vi "KalmanFilterExample.vi"() -> ()   [LabVIEW 2016]
uses:
  <vilib>/addons/Control Design/_Stochastic Systems/Stochastic Systems.llb/Stochastic Systems SubVIs/cd_Stochastic State-Space Model.ctl
  <vilib>/Simulation/Estimation/Implementation/NILVSim Discrete Kalman Filter.llb/SIM Disc KF Pred and Corr with Pred Gain with Checking Direct LV.vi
  <vilib>/Simulation/Implementation/XNodeFramework/SimXNode/SimX.xnode
  <vilib>/addons/Control Design/_Stochastic Systems/NI_CD_Stochastic Systems.lvlib
panel:
  in  "Numeric 2":dbl=5.0 format="%#_13g"
  out "Waveform Chart 2":dbl[](graph)
  out "Waveform Chart":dbl[](graph)
  out "Numeric":i32
  out "Corrected State Estimate xhat(k|k)":dbl[](array[numeric])
  out "Estimated Output yhat(k)":dbl[](array[numeric])
  out "error out":errorcluster
  in  "stop":bool
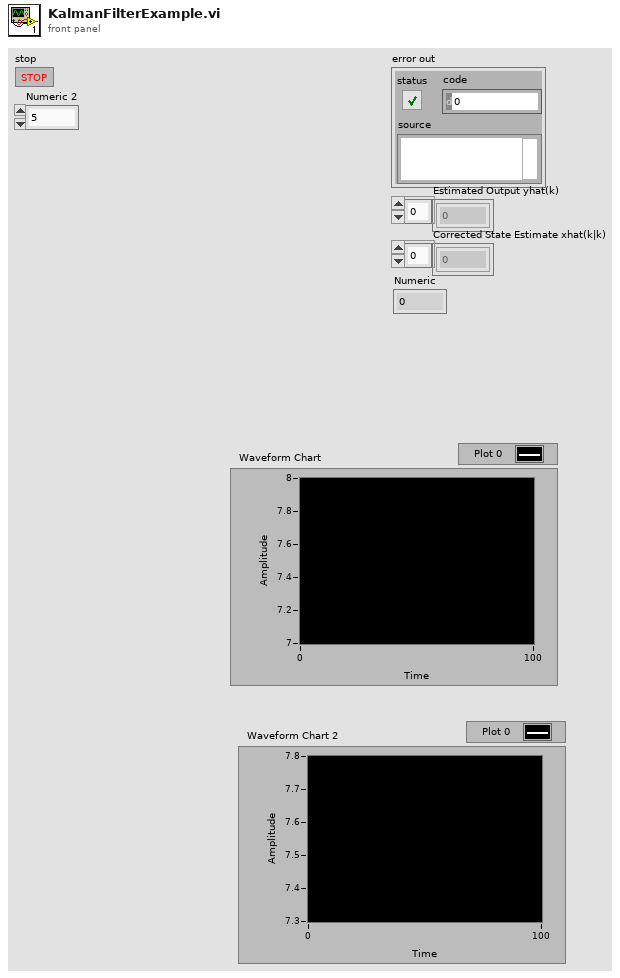
[diagram p1: front panel]
types:
  T1 = typedef "NI_CD_Stochastic Systems.lvlib/cd_Stochastic State-Space Model.ctl" = cluster{"Sampling Time (s)":dbl, "G":dbl[][], "B":dbl[][], "A":dbl[][], "C":dbl[][], "D":dbl[][], "H":dbl[][]}
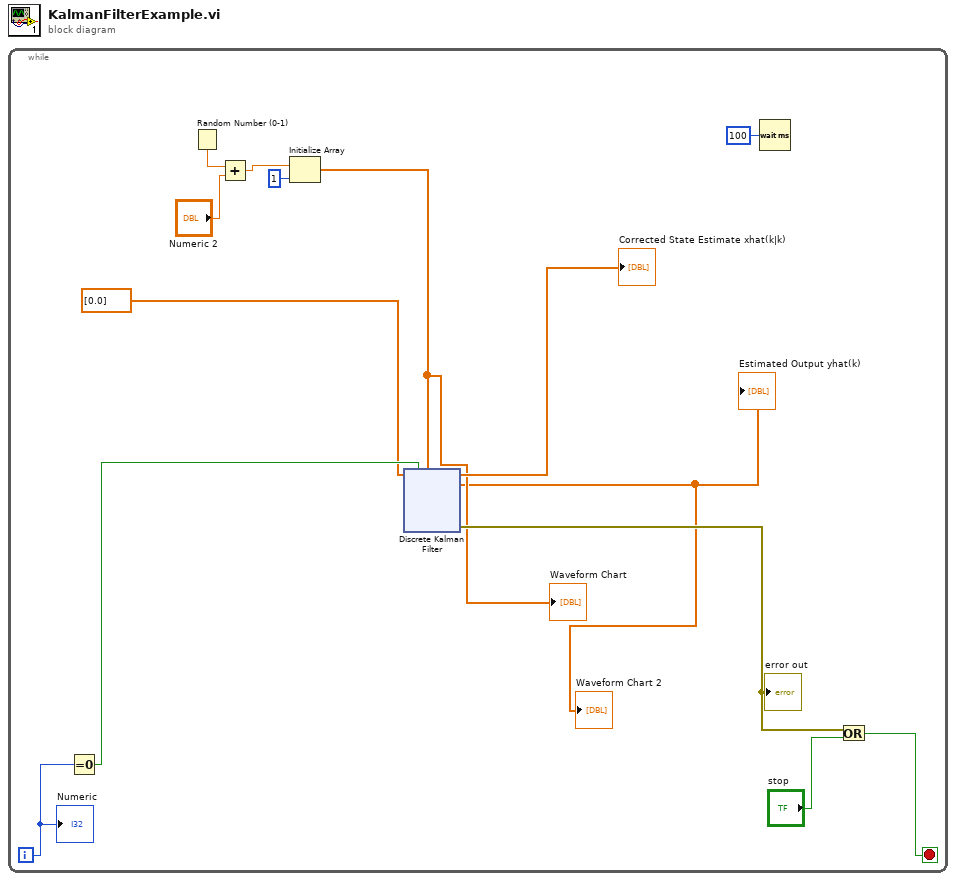
[diagram p0: block diagram]
diagram:
  n1 = while {
    i -> [w11]
    stop <- w10 stop-if-true
    n2 = Equal To 0?(x=w11) -> (x = 0?=w7:bool)
    n3 = Random Number (0-1)() -> (number: 0 to 1=w14:dbl)
    n4 = Add(x=w14, y="Numeric 2") -> (x+y=w12:dbl)
    n5 = Initialize Array(w12, 1 ("dimension size")) -> (w2:dbl[])
    "Waveform Chart" <- w2
    n6 = xnode "Discrete Kalman Filter"("input u(k)"=dbl[] [0.0], "Initialize?"=w7, "Output y(k)"=w2) -> ("Estimated Output yhat(k)"=→"Estimated Output yhat(k)" →"Waveform Chart 2":dbl[], "Corrected State Estimate xhat(k|k)"=→"Corrected State Estimate xhat(k|k)":dbl[], "error out"=w8:errorcluster)  [unwired: 1 in, 5 out]
    "error out" <- w8
    n7 = Wait (ms)(milliseconds to wait=u32 100) -> ()  [unwired: 1 out]
    n8 = Or(x=w8, y="stop") -> (x .or. y?=w10:bool)
    "Numeric" <- w11
  }
